vi "Test Trim String.vi"() -> ()   [LabVIEW 2021]
uses:
  <vilib>/Utility/error.llb/Trim Whitespace.vi
  DataTypes_CIF_U.lvlib
panel:
  out "Pass":bool
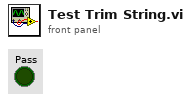
[diagram p1: front panel]
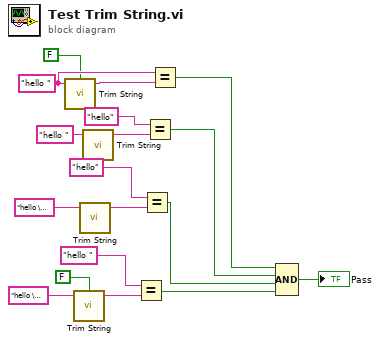
[diagram p0: block diagram]
diagram:
  w11 = "hello " ("String in")
  n1 = call "Trim String.vi"("String in"=w11, "Remove White Space"=FALSE) -> ("Trimmed String"=w12:string)  [unwired: 3 in]
  n2 = call "Trim String.vi"("String in"="hello \u0000", "Remove White Space"=FALSE) -> ("Trimmed String"=w3:string)  [unwired: 3 in]
  n3 = call "Trim String.vi"("String in"="hello \u0000") -> ("Trimmed String"=w9:string)  [unwired: 4 in]
  n4 = call "Trim String.vi"("String in"="hello ") -> ("Trimmed String"=w14:string)  [unwired: 4 in]
  n5 = Equal?(x="hello " ("String in"), y=w3) -> (x = y?=w1:bool)
  n6 = Equal?(x="hello" ("String in"), y=w9) -> (x = y?=w6:bool)
  n7 = Equal?(x="hello" ("String in"), y=w14) -> (x = y?=w17:bool)
  n8 = Equal?(x=w11, y=w12) -> (x = y?=w16:bool)
  n9 = Compound Arithmetic op=AND(w16, w17, w6, w1) -> (→"Pass":bool)
